vi "vehicle.vi"() -> ()   [LabVIEW 2017, in "Class.lvclass"]
uses:
  Class.lvclass
  Class.lvclass/Class.ctl
panel:
  out "Class.lvclass 3":refnum<class "Class.lvclass">
  in  "Class.lvclass":refnum<class "Class.lvclass">
  in  "Interior cargo capacity":dbl=13.1
  in  "model":string="car"
  in  "make":string="Company A"
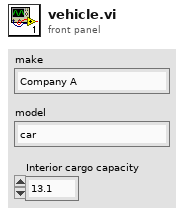
[diagram p1: front panel]
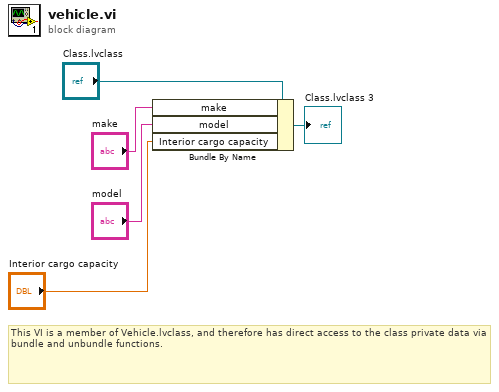
[diagram p0: block diagram]
diagram:
  # "This VI is a member of Vehicle.lvclass, and therefore has direct access to the class private data via bundle and unbundle functions."
  n1 = Bundle By Name(cluster="Class.lvclass", "make"="make", "model"="model", "Interior cargo capacity"="Interior cargo capacity") -> (→"Class.lvclass 3":refnum<class "Class.lvclass">)
